vi "Fit SC Hall.vi"(9 "Flatness":dbl=0.05, 10 "Hall signal":dbl[](array[numeric]), 11 "Field":dbl[](array[numeric])) -> (2 "XY Graph":cluster{"Field":dbl[], dbl[]}[](graph), 3 "Mean":dbl)   [LabVIEW 2018]
uses:
  <vilib>/Analysis/baseanly.llb/Mean (DBL).vi
  <vilib>/Analysis/NI_AALBase.lvlib
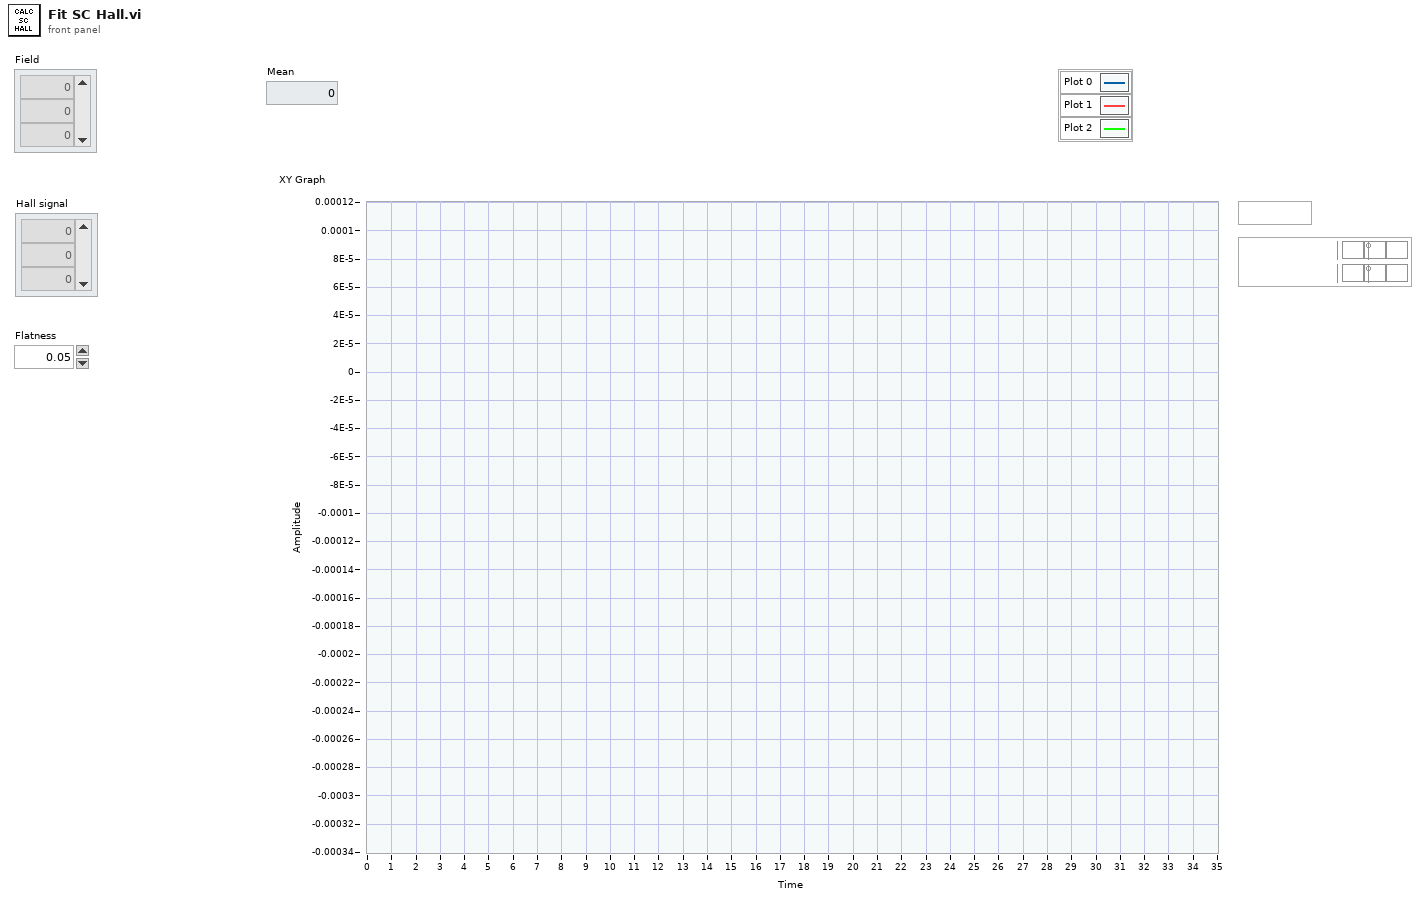
[diagram p1: front panel]
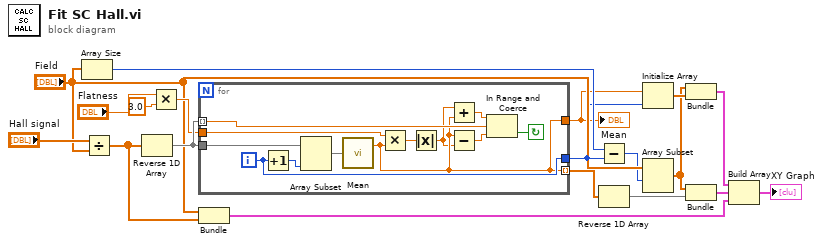
[diagram p0: block diagram]
diagram:
  n1 = Array Size(array="Field") -> (size(s)=w7:i32)
  n2 = Divide(x="Hall signal", y="Field") -> (x/y=w18:dbl[])
  n3 = Reverse 1D Array(array=w18) -> (reversed array=w17:dbl[])
  n4 = Multiply(x="Flatness", y=3.0) -> (x*y=w9:dbl)
  n5 = for {
    tunnel: w17 -> [w28] mode=indexing
    tunnel: w17 -> [w31]
    tunnel: [w21] -> w16 mode=indexing
    tunnel: w9 -> [w23]
    tunnel: [w24] -> w1
    tunnel: [w21] -> w6
    i -> [w24]
    stop <- w25 continue-if-true
    n6 = Increment(x=w24) -> (x+1=w30:i32)
    n7 = Array Subset(array=w31, length=w30) -> (w29:dbl[])  [unwired: 1 in]
    n8 = call-poly <vilib>:"Mean.vi"("X"=w29) -> ("mean"=w21:dbl)  [unwired: 1 out]
    n9 = Multiply(x=w23, y=w21) -> (x*y=w22:dbl)
    n10 = Absolute Value(x=w22) -> (abs(x)=w20:dbl)
    n11 = Add(x=w20, y=w21) -> (x+y=w27:dbl)
    n12 = Subtract(x=w21, y=w20) -> (x-y=w26:dbl)
    n13 = In Range and Coerce(upper limit=w27, x=w28, lower limit=w26) -> (In Range?=w25:bool)  [unwired: 1 out]
  }
  "Mean" <- w6
  n14 = Bundle("Field"="Field", w18) -> (w13:cluster{"Field":dbl[], dbl[]})  [unwired: 1 in]
  n15 = Subtract(x=w7, y=w1) -> (x-y=w5:i32)
  n16 = Reverse 1D Array(array=w16) -> (reversed array=w15:dbl[])
  n17 = Initialize Array(w6, w1) -> (w4:dbl[])
  n18 = Array Subset(array="Field", index=w5) -> (w3:dbl[])  [unwired: 1 in]
  n19 = Bundle(w3, w4) -> (w2:cluster{dbl[], dbl[]})  [unwired: 1 in]
  n20 = Bundle(w3, w15) -> (w12:cluster{dbl[], dbl[]})  [unwired: 1 in]
  n21 = Build Array(w2, w12, w13) -> (→"XY Graph":cluster{"Field":dbl[], dbl[]}[])
